vi "StartSubRoutine.vi"(11 "GeneralAutoInput":T1) -> (1 "Okay to start?":bool, 2 "Local Start":timestamp, 3 "End by:":timestamp, 4 "Auto Start Time":timestamp)   [LabVIEW 2017]
uses:
  AutoSubsystem/AutoInput.ctl
  AutoSubsystem/AutoSubroutine.lvclass
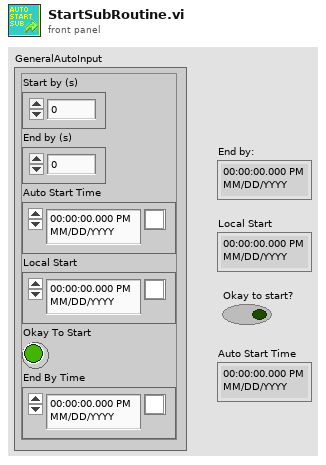
[diagram p1: front panel]
types:
  T1 = typedef "AutoSubroutine.lvclass/AutoInput.ctl" = cluster{"Start by (s)":dbl, "End by (s)":dbl, "Auto Start Time":timestamp, "Local Start":timestamp, "Okay To Start":bool, "End By Time":timestamp}
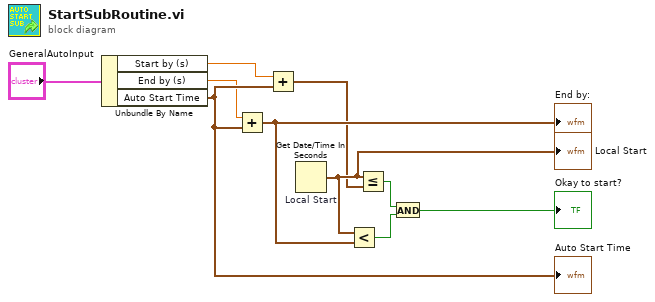
[diagram p0: block diagram]
diagram:
  n1 = Unbundle By Name("GeneralAutoInput") -> ("Start by (s)"=w1:dbl, "End by (s)"=w3:dbl, "Auto Start Time"=w10:timestamp)
  "Auto Start Time" <- w10
  n2 = Add(x=w3, y=w10) -> (x+y=w5:timestamp)
  "End by:" <- w5
  n3 = Add(x=w1, y=w10) -> (x+y=w4:timestamp)
  n4 = Get Date/Time In Seconds "Local Start"() -> (seconds since 1Jan1904=w9:timestamp)
  "Local Start" <- w9
  n5 = Less?(x=w9, y=w5) -> (x < y?=w7:bool)
  n6 = Less Or Equal?(x=w9, y=w4) -> (x <= y?=w6:bool)
  n7 = And(x=w6, y=w7) -> (x .and. y?=→"Okay to start?":bool)
